vi "Get Session Property (Core).vi"(0 "SLSC Local in":refnum<class "SLSC Local.lvclass">, 11 "error in (no error)":errorcluster) -> (4 "SLSC Local out":refnum<class "SLSC Local.lvclass">, 15 "error out":errorcluster)   [LabVIEW 2015]
uses:
  SLSC Local.lvclass
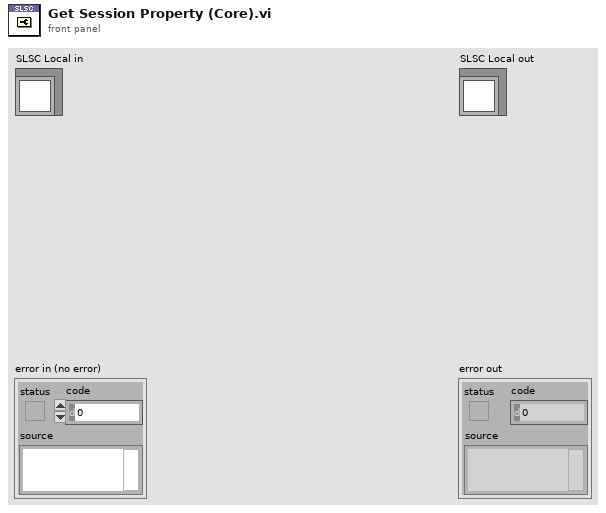
[diagram p1: front panel]
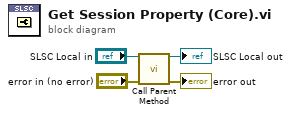
[diagram p0: block diagram]
diagram:
  n1 = call-parent "Call Parent Method"("SLSC Interface in"="SLSC Local in", "error in (no error)"="error in (no error)") -> ("SLSC Interface out"=→"SLSC Local out":refnum<class "SLSC Local.lvclass">, "error out"=→"error out":errorcluster)  [unwired: 12 in]
